vi "RawModbus_To_Data.vi"(8 "ErrorIn":errorcluster, 10 "InpuData":u16[](array[numeric]), 11 "Read Data Type":enum16{"String", "Intiger", "DBL", "SGL"}(ring)) -> (0 "ErrorOut":errorcluster, 1 "Array":sgl[](array[numeric]), 2 "16bit integer":i16[](array[numeric]), 3 "String":string)   [LabVIEW 2024]
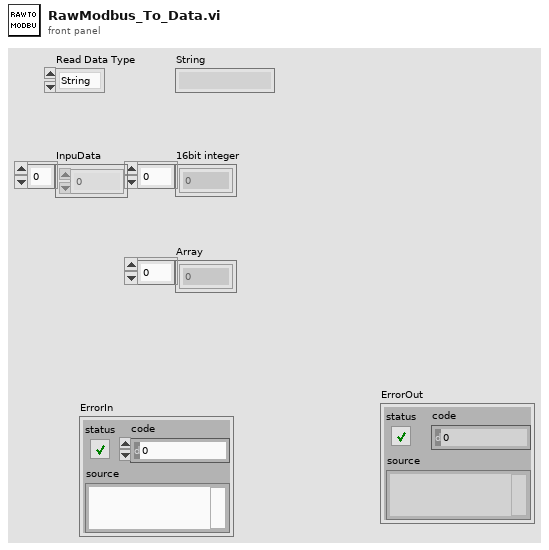
[diagram p1: front panel]
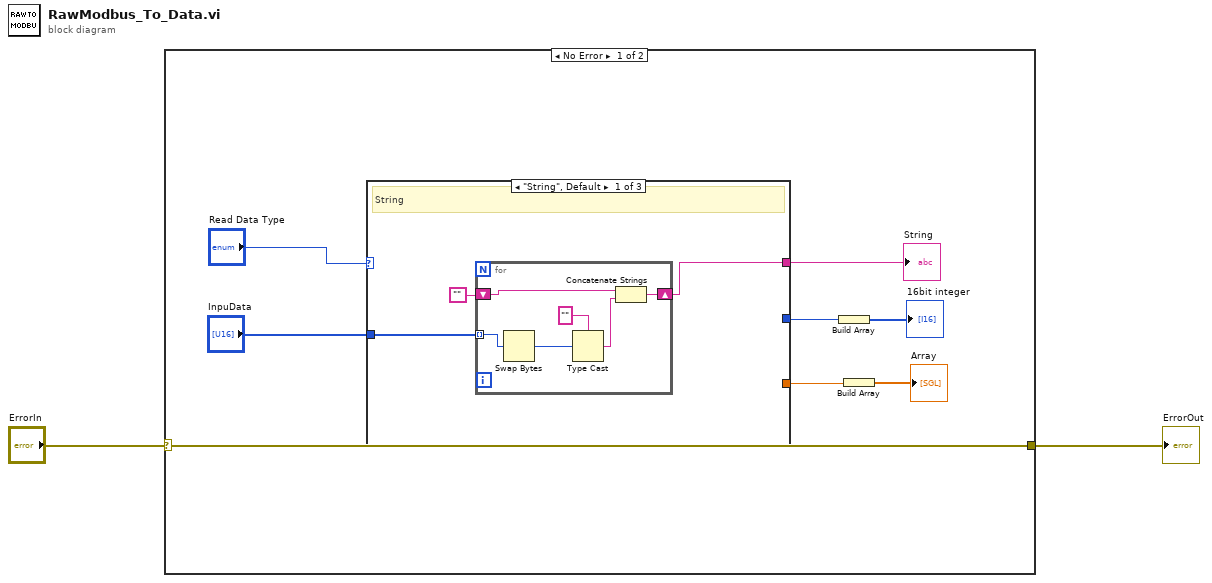
[diagram p0: block diagram]
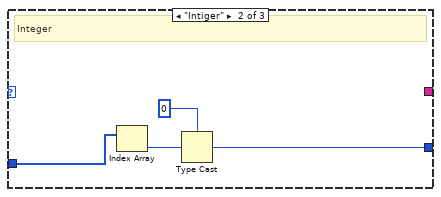
[diagram p2: hidden frame]
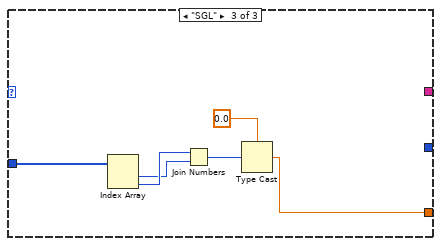
[diagram p3: hidden frame]
diagram:
  n1 = case shown="No Error" "ErrorIn" {
    selector: "ErrorIn" -> [w7 w30]
    tunnel: [w7 w30] -> w1
    frame No Error {
      n2 = case shown="\"String\", Default" "Read Data Type" {
        tunnel: "InpuData" -> [w12 w20 w27]
        tunnel: [w11 _ _] -> w10
        tunnel: [_ w21 _] -> w4
        tunnel: [_ _ w24] -> w6
        frame "String", Default {
          # "String"
          n3 = for {
            shift-right: [w18] -> w11
            shift-left: "" -> [w16]
            tunnel: w12 -> [w14] mode=indexing
            n4 = Swap Bytes(anything=w14) -> (byte swapped=w15:u16)
            n5 = Type Cast(type="", x=w15) -> (*(type *) &x=w17:string)
            n6 = Concatenate Strings(w16, w17) -> (w18:string)
          }
        }
        frame "Intiger" {
          # "Integer"
          n7 = Index Array(array=w20) -> (element=w23:u16)  [unwired: 1 in]
          n8 = Type Cast(type=i16 0 ("16bit integer"), x=w23) -> (*(type *) &x=w21:i16)
        }
        frame "SGL" {
          n9 = Index Array(array=w27) -> (element #1=w25:u16, element #2=w26:u16)  [unwired: 2 in]
          n10 = Join Numbers(hi=w26, lo=w25) -> ((hi.lo)=w29:u32)
          n11 = Type Cast(type=sgl 0.0, x=w29) -> (*(type *) &x=w24:sgl)
        }
      }
      "String" <- w10
      n12 = Build Array(w4) -> (→"16bit integer":i16[])
      n13 = Build Array(w6) -> (→"Array":sgl[])
    }
    frame Error {
    }
  }
  "ErrorOut" <- w1
